vi "Principal.vi"() -> ()   [LabVIEW 2018]
uses:
  <vilib>/LabVIEW Interface for Arduino/Type Defs/Arduino Resource.ctl
  <vilib>/LabVIEW Interface for Arduino/Type Defs/Board Type.ctl
  <vilib>/LabVIEW Interface for Arduino/Type Defs/Connection Type.ctl
  <vilib>/LabVIEW Interface for Arduino/Type Defs/Pin Mode.ctl
  <vilib>/LabVIEW Interface for Arduino/LabVIEW Interface for Arduino.lvlib
panel:
  out "Mensagem":string
  in  "ATUALIZAR CAP":bool=TRUE
  in  "index":i32
  out "CAL":bool=TRUE
  out "Arduino Resource out":T3
  out "BT_Endereco":string[](array[string])
  out "BT_Nome":string[](array[string])
  in  "Frames":enum32{"Menu", "Medição", "Calibração"}(tab)
  in  "SAIR":bool
  in  "Atualizar":bool
  in  "Dispositivos Encontrados":i32(listbox)
  in  "Conectar":bool
  in  "Cap Ext.":bool
  in  "Resitor:":u32=4700 format="%.0f Ohms"
  in  "SAIR 2":bool
  in  "Capacitor:":dbl=0.8 min=0.0 max=408.8 step=0.8 format="%.2f uF"
  in  "LER CAPACITOR":bool
  out "Valor Lido:":dbl format="%.2f uF"
  in  "STOP CAL":bool
  out "Table":string[][](table)
  in  "CALIBRA敲O":bool
  out "Tempo Estimado (s)":dbl
  out "Pontos Lidos":dbl
  out "Pontos Restante":dbl
  out "Arduino Resource":T4={"VISA resource"="", "Board Type"=enum."Uno", "Connection Type"=enum."USB / Serial", "Bytes Per Packet (15)"=15}
  # "V2.1"
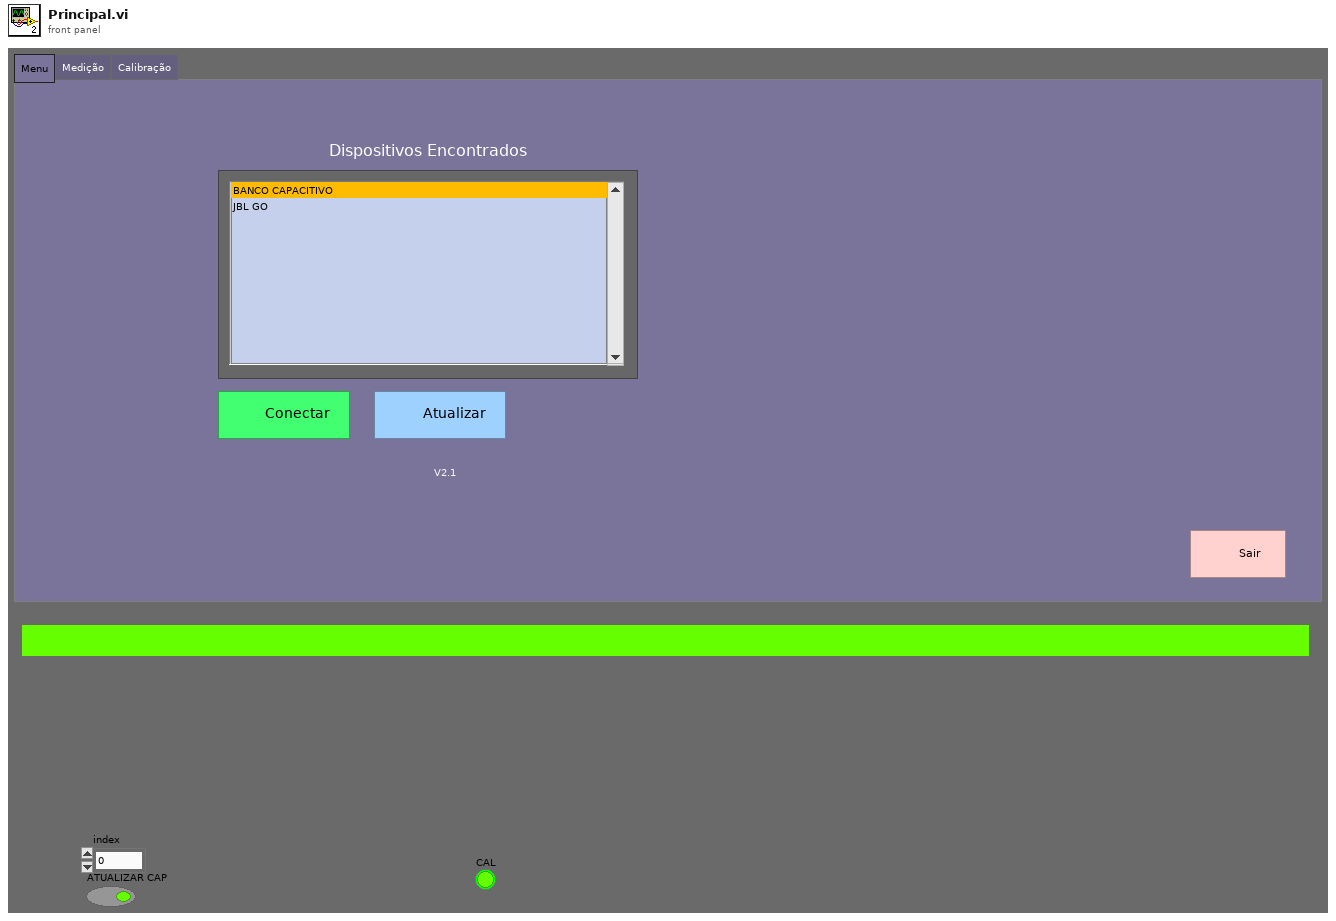
[diagram p1: front panel]
types:
  T1 = typedef "LabVIEW Interface for Arduino.lvlib/Board Type.ctl" = enum16{"Uno", "Dimuelanove w/Atmega 328", "Mega 2560"}
  T2 = typedef "LabVIEW Interface for Arduino.lvlib/Connection Type.ctl" = enum8{"USB / Serial", "XBEE", "BlueSmirf (Bluetooth)"}
  T3 = cluster{"connection ID in":refnum<k31>, "Board Type (Uno)":T1, "Connection Type (USB/Serial)":T2, "Bytes Per Packet (15)":u32}
  T4 = typedef "LabVIEW Interface for Arduino.lvlib/Arduino Resource.ctl" = cluster{"VISA resource":refnum<visa-resource-name>, "Board Type":T1, "Connection Type":enum8{"USB / Serial"}, "Bytes Per Packet (15)":u8}
  T5 = typedef "LabVIEW Interface for Arduino.lvlib/Pin Mode.ctl" = enum8{"Input", "Output"}
  T6 = cluster{"Address":string, "Device Name":string}[]
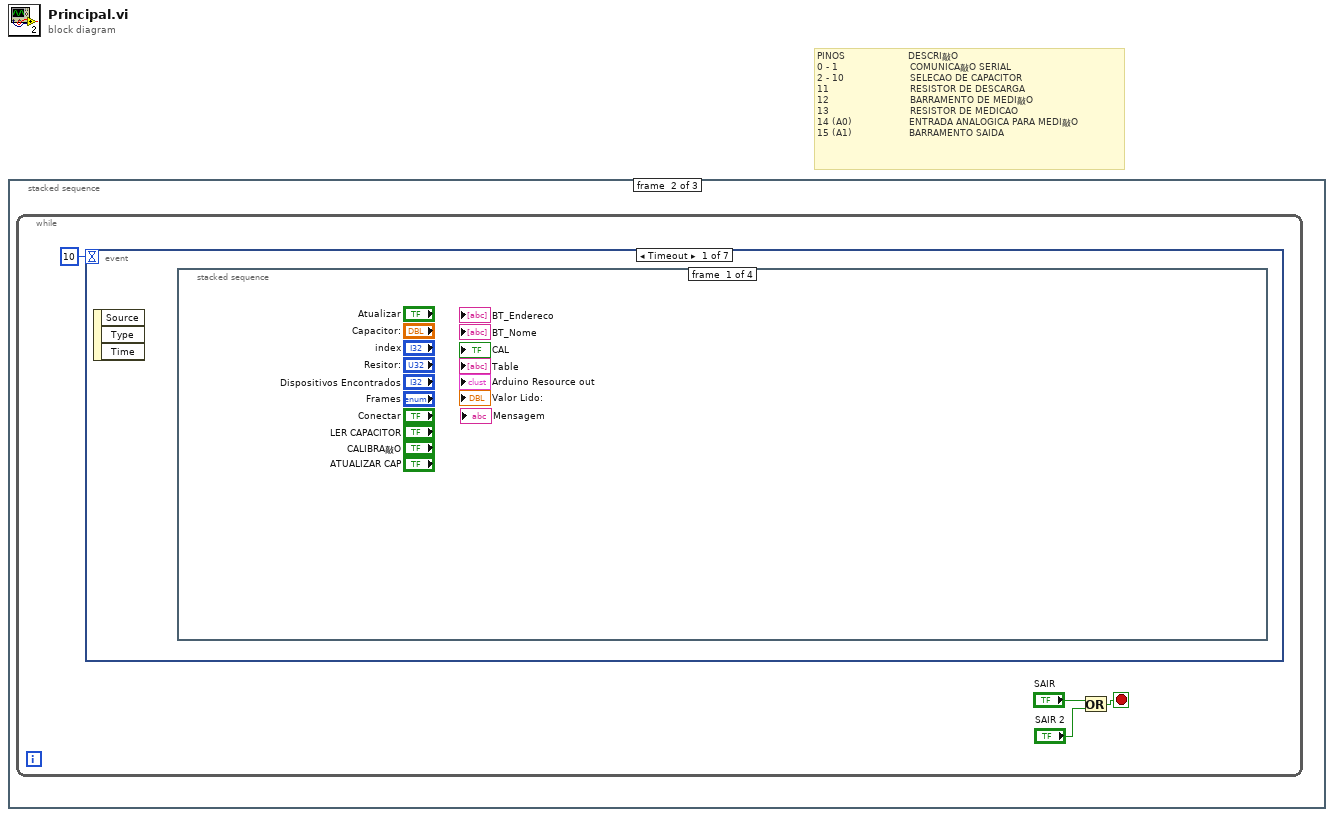
[diagram p0: block diagram]
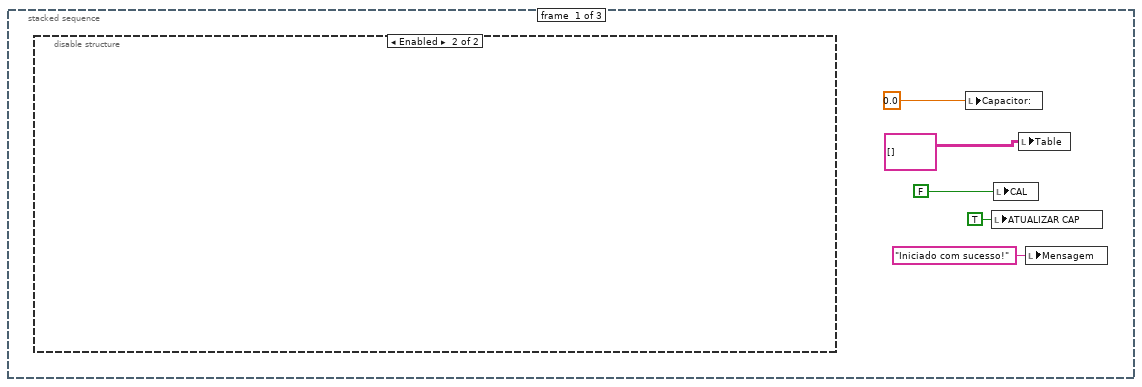
[diagram p2: hidden frame]
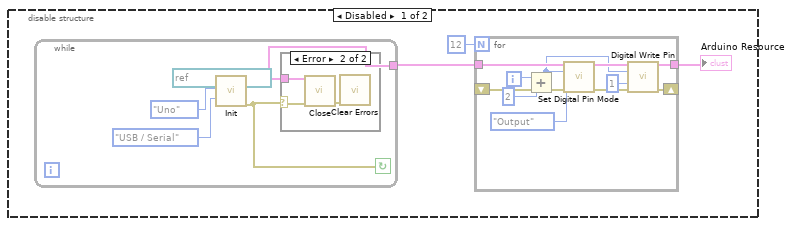
[diagram p3: hidden frame]
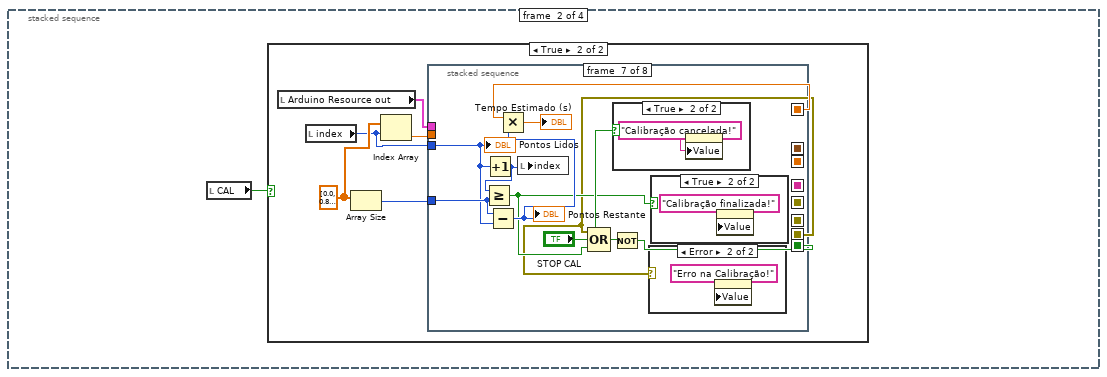
[diagram p5: hidden frame]
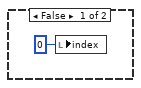
[diagram p6: hidden frame]
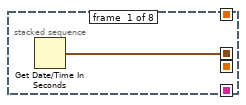
[diagram p7: hidden frame]
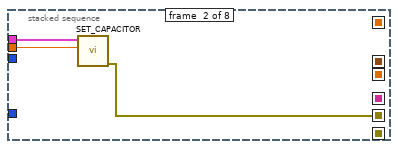
[diagram p8: hidden frame]
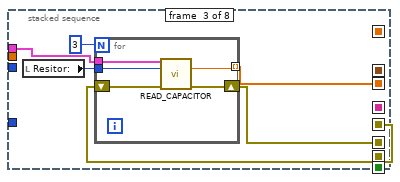
[diagram p9: hidden frame]
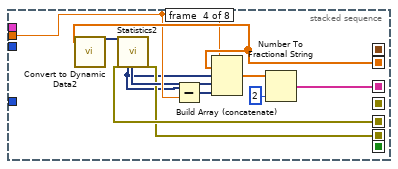
[diagram p10: hidden frame]
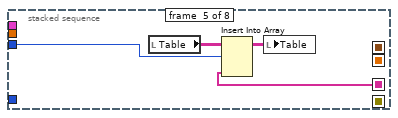
[diagram p11: hidden frame]
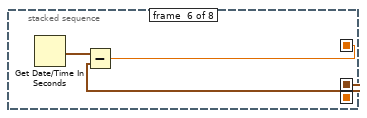
[diagram p12: hidden frame]
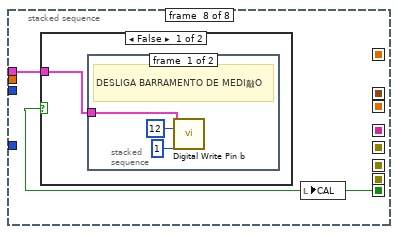
[diagram p16: hidden frame]
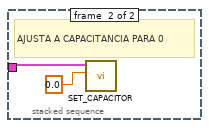
[diagram p17: hidden frame]
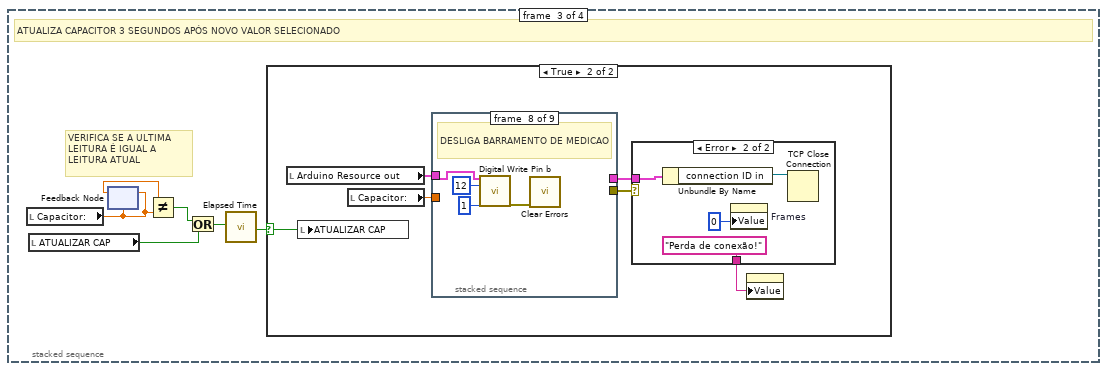
[diagram p19: hidden frame]
diagram:
  # "PINOS                     DESCRI敲O\n0 - 1                        COMUNICA敲O SERIAL\n2 - 10                      SELECAO DE CAPACITOR\n11                           RESISTOR DE DESCARGA\n12                           BARRAMENTO DE MEDI敲O\n13                           RESISTOR DE MEDICAO\n14 (A0)                   ENTRADA ANALOGICA PARA MEDI敲O\n15 (A1)                   BARRAMENTO SAIDA"
  n1 = stacked-sequence {
    frame #0 {
      n2 = disable-structure shown="Enabled" {
        frame Disabled {
          n3 = while {
            tunnel: [w21] -> w7
            stop <- w22 continue-if-true
            n4 = call <vilib>:"Init.vi"("VISA resource"=refnum<visa-resource-name> "ASRL8::INSTR", "Board Type (Uno)"=Board_Type."Uno", "Connection Type (USB/Serial)"=Connection_Type."USB / Serial") -> ("Arduino Resource"=w21:T4, "error out"=w22:errorcluster)  [unwired: 15 in]
            n5 = case shown="Error" w22 {
              selector: w22 -> [_ w26]
              tunnel: w21 -> [_ w27]
              frame No Error {
              }
              frame Error {
                n6 = call <vilib>:"Close.vi"("Arduino Resource"=w27, "error in"=w26) -> ("error out"=w25:errorcluster)  [unwired: 13 in]
                n7 = call <vilib>:"Clear Errors.vi"("error in (no error)"=w25) -> ()  [unwired: 5 in, 2 out]
              }
            }
          }
          n8 = for {
            N: 12 -> [_]
            tunnel: w7 -> [w19]
            shift-right: [w14] -> _
            shift-left: _ -> [w17]
            tunnel: [w13] -> w8
            i -> [w12]
            n9 = Add(x=w12, y=2) -> (x+y=w11:i32)
            n10 = call <vilib>:"Set Digital Pin Mode.vi"("Arduino Resource"=w19, "Digital I/O Pin"=w11, "Pin Mode (Input)"=Pin_Mode."Output", "error in"=w17) -> ("Arduino Resource"=w16:T4, "error out"=w15:errorcluster)  [unwired: 10 in]
            n11 = call <vilib>:"Digital Write Pin.vi"("Arduino Resource"=w16, "Digital I/O Pin (0)"=w11, "Value (0)"=u8 1, "error in"=w15) -> ("Arduino Resource"=w13:T4, "error out"=w14:errorcluster)  [unwired: 10 in]
          }
          "Arduino Resource" <- w8
        }
        frame Enabled {
        }
      }
      n12 = local write "Capacitor:"(0.0 ("Capacitor")) -> ()
      n13 = local write "ATUALIZAR CAP"(TRUE ("ATUALIZAR CAP")) -> ()
      n14 = local write "CAL"(FALSE ("CAL")) -> ()
      n15 = local write "Table"(string[][] [] ("Table")) -> ()
      n16 = local write "Mensagem"("Iniciado com sucesso!" ("Mensagem")) -> ()
    }
    frame #1 {
      n17 = while {
        stop <- w28 stop-if-true
        n18 = event shown="[0] Timeout" {
          selector: _ -> [_ _ _ _ _ _ _]
          dyn-events: _ -> [_ _ _ _ _ _ _]
          timeout: 10 -> [_ _ _ _ _ _ _]
          event Timeout {
            n19 = event-data() -> ()  [unwired: 1 in, 3 out]
            n20 = stacked-sequence {
              frame #0 {
              }
              frame #1 {
                n21 = local read "CAL"() -> (w32:bool)
                n22 = case shown="True" w32 {
                  frame False {
                    n23 = local write "index"(0 ("index")) -> ()
                  }
                  frame True {
                    w37 = dbl[] [0.0, 0.8, 1.6, 2.4000000000000004, 3.2, 4.0, 4.8, 5.6, 6.3999999999999995, 7.199999999999999, 7.999999999999999, 8.799999999999999, 9.6, 10.4, 11.200000000000001, 12.000000000000002, 12.800000000000002, 13.600000000000003, 14.400000000000004, 15.200000000000005, 16.000000000000004, 16.800000000000004, 17.600000000000005, 18.400000000000006, 19.200000000000006, 20.000000000000007, 20.800000000000008, 21.60000000000001, 22.40000000000001, 23.20000000000001, 24.00000000000001, 24.80000000000001, 25.600000000000012, 26.400000000000013, 27.200000000000014, 28.000000000000014, 28.800000000000015, 29.600000000000016, 30.400000000000016, 31.200000000000017, 32.000000000000014, 32.80000000000001, 33.60000000000001, 34.400000000000006, 35.2, 36.0, 36.8, 37.599999999999994, 38.39999999999999, 39.19999999999999, 39.999999999999986, 40.79999999999998, 41.59999999999998, 42.39999999999998, 43.199999999999974, 43.99999999999997, 44.79999999999997, 45.599999999999966, 46.39999999999996, 47.19999999999996, 47.99999999999996, 48.799999999999955, 49.59999999999995, 50.39999999999995, 51.199999999999946, 51.99999999999994, 52.79999999999994, 53.59999999999994, 54.399999999999935, 55.19999999999993, 55.99999999999993, 56.799999999999926, 57.59999999999992, 58.39999999999992, 59.19999999999992, 59.999999999999915, 60.79999999999991, 61.59999999999991, 62.399999999999906, 63.1999999999999, 63.9999999999999, 64.7999999999999, 65.5999999999999, 66.39999999999989, 67.19999999999989, 67.99999999999989, 68.79999999999988, 69.59999999999988, 70.39999999999988, 71.19999999999987, 71.99999999999987, 72.79999999999987, 73.59999999999987, 74.39999999999986, 75.19999999999986, 75.99999999999986, 76.79999999999986, 77.59999999999985, 78.39999999999985, 79.19999999999985, 79.99999999999984, 80.79999999999984, 81.59999999999984, 82.39999999999984, 83.19999999999983, 83.99999999999983, 84.79999999999983, 85.59999999999982, 86.39999999999982, 87.19999999999982, 87.99999999999982, 88.79999999999981, 89.59999999999981, 90.3999999999998, 91.1999999999998, 91.9999999999998, 92.7999999999998, 93.5999999999998, 94.39999999999979, 95.19999999999979, 95.99999999999979, 96.79999999999978, 97.59999999999978, 98.39999999999978, 99.19999999999978, 99.99999999999977, 100.79999999999977, 101.59999999999977, 102.39999999999976, 103.19999999999976, 103.99999999999976, 104.79999999999976, 105.59999999999975, 106.39999999999975, 107.19999999999975, 107.99999999999974, 108.79999999999974, 109.59999999999974, 110.39999999999974, 111.19999999999973, 111.99999999999973, 112.79999999999973, 113.59999999999972, 114.39999999999972, 115.19999999999972, 115.99999999999972, 116.79999999999971, 117.59999999999971, 118.39999999999971, 119.1999999999997, 119.9999999999997, 120.7999999999997, 121.5999999999997, 122.3999999999997, 123.19999999999969, 123.99999999999969, 124.79999999999968, 125.59999999999968, 126.39999999999968, 127.19999999999968, 127.99999999999967, 128.79999999999967, 129.59999999999968, 130.3999999999997, 131.1999999999997, 131.99999999999972, 132.79999999999973, 133.59999999999974, 134.39999999999975, 135.19999999999976, 135.99999999999977, 136.79999999999978, 137.5999999999998, 138.3999999999998, 139.19999999999982, 139.99999999999983, 140.79999999999984, 141.59999999999985, 142.39999999999986, 143.19999999999987, 143.9999999999999, 144.7999999999999, 145.5999999999999, 146.39999999999992, 147.19999999999993, 147.99999999999994, 148.79999999999995, 149.59999999999997, 150.39999999999998, 151.2, 152.0, 152.8, 153.60000000000002, 154.40000000000003, 155.20000000000005, 156.00000000000006, 156.80000000000007, 157.60000000000008, 158.4000000000001, 159.2000000000001, 160.0000000000001, 160.80000000000013, 161.60000000000014, 162.40000000000015, 163.20000000000016, 164.00000000000017, 164.80000000000018, 165.6000000000002, 166.4000000000002, 167.20000000000022, 168.00000000000023, 168.80000000000024, 169.60000000000025, 170.40000000000026, 171.20000000000027, 172.00000000000028, 172.8000000000003, 173.6000000000003, 174.40000000000032, 175.20000000000033, 176.00000000000034, 176.80000000000035, 177.60000000000036, 178.40000000000038, 179.2000000000004, 180.0000000000004, 180.8000000000004, 181.60000000000042, 182.40000000000043, 183.20000000000044, 184.00000000000045, 184.80000000000047, 185.60000000000048, 186.4000000000005, 187.2000000000005, 188.0000000000005, 188.80000000000052, 189.60000000000053, 190.40000000000055, 191.20000000000056, 192.00000000000057, 192.80000000000058, 193.6000000000006, 194.4000000000006, 195.2000000000006, 196.00000000000063, 196.80000000000064, 197.60000000000065, 198.40000000000066, 199.20000000000067, 200.00000000000068, 200.8000000000007, 201.6000000000007, 202.40000000000072, 203.20000000000073, 204.00000000000074, 204.80000000000075, 205.60000000000076, 206.40000000000077, 207.20000000000078, 208.0000000000008, 208.8000000000008, 209.60000000000082, 210.40000000000083, 211.20000000000084, 212.00000000000085, 212.80000000000086, 213.60000000000088, 214.4000000000009, 215.2000000000009, 216.0000000000009, 216.80000000000092, 217.60000000000093, 218.40000000000094, 219.20000000000095, 220.00000000000097, 220.80000000000098, 221.600000000001, 222.400000000001, 223.200000000001, 224.00000000000102, 224.80000000000103, 225.60000000000105, 226.40000000000106, 227.20000000000107, 228.00000000000108, 228.8000000000011, 229.6000000000011, 230.4000000000011, 231.20000000000113, 232.00000000000114, 232.80000000000115, 233.60000000000116, 234.40000000000117, 235.20000000000118, 236.0000000000012, 236.8000000000012, 237.60000000000122, 238.40000000000123, 239.20000000000124, 240.00000000000125, 240.80000000000126, 241.60000000000127, 242.40000000000128, 243.2000000000013, 244.0000000000013, 244.80000000000132, 245.60000000000133, 246.40000000000134, 247.20000000000135, 248.00000000000136, 248.80000000000138, 249.6000000000014, 250.4000000000014, 251.2000000000014, 252.00000000000142, 252.80000000000143, 253.60000000000144, 254.40000000000146, 255.20000000000147, 256.0000000000015, 256.8000000000015, 257.6000000000015, 258.4000000000015, 259.2000000000015, 260.00000000000153, 260.80000000000155, 261.60000000000156, 262.40000000000157, 263.2000000000016, 264.0000000000016, 264.8000000000016, 265.6000000000016, 266.4000000000016, 267.20000000000164, 268.00000000000165, 268.80000000000166, 269.60000000000167, 270.4000000000017, 271.2000000000017, 272.0000000000017, 272.8000000000017, 273.6000000000017, 274.40000000000174, 275.20000000000175, 276.00000000000176, 276.8000000000018, 277.6000000000018, 278.4000000000018, 279.2000000000018, 280.0000000000018, 280.80000000000183, 281.60000000000184, 282.40000000000185, 283.20000000000186, 284.0000000000019, 284.8000000000019, 285.6000000000019, 286.4000000000019, 287.2000000000019, 288.00000000000193, 288.80000000000194, 289.60000000000196, 290.40000000000197, 291.200000000002, 292.000000000002, 292.800000000002, 293.600000000002, 294.400000000002, 295.20000000000203, 296.00000000000205, 296.80000000000206, 297.60000000000207, 298.4000000000021, 299.2000000000021, 300.0000000000021, 300.8000000000021, 301.6000000000021, 302.40000000000214, 303.20000000000215, 304.00000000000216, 304.80000000000217, 305.6000000000022, 306.4000000000022, 307.2000000000022, 308.0000000000022, 308.8000000000022, 309.60000000000224, 310.40000000000225, 311.20000000000226, 312.0000000000023, 312.8000000000023, 313.6000000000023, 314.4000000000023, 315.2000000000023, 316.00000000000233, 316.80000000000234, 317.60000000000235, 318.40000000000236, 319.2000000000024, 320.0000000000024, 320.8000000000024, 321.6000000000024, 322.4000000000024, 323.20000000000243, 324.00000000000244, 324.80000000000246, 325.60000000000247, 326.4000000000025, 327.2000000000025, 328.0000000000025, 328.8000000000025, 329.6000000000025, 330.40000000000254, 331.20000000000255, 332.00000000000256, 332.80000000000257, 333.6000000000026, 334.4000000000026, 335.2000000000026, 336.0000000000026, 336.8000000000026, 337.60000000000264, 338.40000000000265, 339.20000000000266, 340.0000000000027, 340.8000000000027, 341.6000000000027, 342.4000000000027, 343.2000000000027, 344.00000000000273, 344.80000000000274, 345.60000000000275, 346.40000000000276, 347.2000000000028, 348.0000000000028, 348.8000000000028, 349.6000000000028, 350.4000000000028, 351.20000000000283, 352.00000000000284, 352.80000000000285, 353.60000000000286, 354.4000000000029, 355.2000000000029, 356.0000000000029, 356.8000000000029, 357.6000000000029, 358.40000000000293, 359.20000000000294, 360.00000000000296, 360.80000000000297, 361.600000000003, 362.400000000003, 363.200000000003, 364.000000000003, 364.800000000003, 365.60000000000304, 366.40000000000305, 367.20000000000306, 368.00000000000307, 368.8000000000031, 369.6000000000031, 370.4000000000031, 371.2000000000031, 372.0000000000031, 372.80000000000314, 373.60000000000315, 374.40000000000316, 375.2000000000032, 376.0000000000032, 376.8000000000032, 377.6000000000032, 378.4000000000032, 379.20000000000323, 380.00000000000324, 380.80000000000325, 381.60000000000326, 382.4000000000033, 383.2000000000033, 384.0000000000033, 384.8000000000033, 385.6000000000033, 386.40000000000333, 387.20000000000334, 388.00000000000335, 388.80000000000337, 389.6000000000034, 390.4000000000034, 391.2000000000034, 392.0000000000034, 392.8000000000034, 393.60000000000343, 394.40000000000344, 395.20000000000346, 396.00000000000347, 396.8000000000035, 397.6000000000035, 398.4000000000035, 399.2000000000035, 400.0000000000035, 400.80000000000354, 401.60000000000355, 402.40000000000356, 403.20000000000357, 404.0000000000036, 404.8000000000036, 405.6000000000036, 406.4000000000036, 407.2000000000036, 408.00000000000364, 408.80000000000365] ("Array")
                    n24 = local read "Arduino Resource out"() -> (w38:T3)
                    n25 = local read "index"() -> (w35:i32)
                    n26 = Array Size(array=w37) -> (size(s)=w34:i32)
                    n27 = Index Array(array=w37, index=w35) -> (element=w36:dbl)
                    n28 = stacked-sequence {
                      seq-local: [w39 _ _ _ _ _ _ _] -> [_ _ _ _ _ w70 _ _]
                      seq-local: [_ _ w45 _ _ _ _ _] -> [_ _ _ w63 _ _ _ _]
                      seq-local: [_ _ _ w60 _ _ _ _] -> [_ _ _ _ w66 _ _ _]
                      seq-local: [_ w40 _ _ _ _ _ _] -> [_ _ w44 _ _ _ _ _]
                      seq-local: [_ _ w43 _ _ _ _ _] -> [_ _ _ w59 _ _ _ _]
                      seq-local: [_ _ _ _ _ w69 _ _] -> [_ _ _ _ _ _ w78 _]
                      seq-local: [_ _ _ w55 _ _ _ _] -> [_ _ _ _ _ _ w73 _]
                      seq-local: [_ _ _ _ _ _ w76 _] -> [_ _ _ _ _ _ _ w87]
                      tunnel: w35 -> [_ _ _ _ w65 _ w80 _]
                      tunnel: w36 -> [_ w41 _ w58 _ _ _ _]
                      tunnel: w38 -> [_ w42 w46 _ _ _ _ w86]
                      tunnel: w34 -> [_ _ _ _ _ _ w81 _]
                      frame #0 {
                        n29 = Get Date/Time In Seconds() -> (seconds since 1Jan1904=w39:timestamp)
                      }
                      frame #1 {
                        n30 = call "SET_CAPACITOR.vi"("Arduino Resource in"=w42, "Capacitor"=w41) -> ("error out"=w40:errorcluster)  [unwired: 7 in, 1 out]
                      }
                      frame #2 {
                        n31 = local read "Resitor:"() -> (w48:u32)
                        n32 = for {
                          N: 3 -> [_]
                          tunnel: w46 -> [w52]
                          tunnel: w48 -> [w51]
                          tunnel: [w50] -> w45 mode=indexing
                          shift-right: [w49] -> w43
                          shift-left: w44 -> [w53]
                          n33 = call "READ_CAPACITOR.vi"("Arduino Resource in"=w52, "Resitor"=w51, "error in"=w53) -> ("Capacitor"=w50:dbl, "error out"=w49:errorcluster)  [unwired: 10 in, 1 out]
                        }
                      }
                      frame #3 {
                        n34 = call "Convert to Dynamic Data2"("Array"=w63) -> ("Dynamic Data Type"=w64:dynamicdata)  [unwired: 3 in]
                        n35 = call "Statistics2"("Signals"=w64, "error in (no error)"=w59) -> ("Median"=w54:dynamicdata, "Standard Dev"=w56:dynamicdata, "error out"=w55:errorcluster)  [unwired: 23 in]
                        n36 = Subtract(x=w54, y=w58) -> (x-y=w57:dynamicdata)
                        n37 = Build Array (concatenate)(w58, w63, w54, w56, w57) -> (w62:dbl[])
                        n38 = Number To Fractional String(number=w62, precision (6)=i16 2) -> (F-format string=w60:string[])  [unwired: 2 in]
                      }
                      frame #4 {
                        n39 = local read "Table"() -> (w68:string[][])
                        n40 = Insert Into Array(array=w68, index (row)=w65, new element=w66) -> (w67:string[][])  [unwired: 1 in]
                        n41 = local write "Table"(w67) -> ()
                      }
                      frame #5 {
                        n42 = Get Date/Time In Seconds() -> (seconds since 1Jan1904=w71:timestamp)
                        n43 = Subtract(x=w71, y=w70) -> (x-y=w69:dbl)
                      }
                      frame #6 {
                        n44 = Increment(x=w80) -> (x+1=w82:i32)
                        n45 = Greater Or Equal?(x=w82, y=w81) -> (x >= y?=w74:bool)
                        n46 = Subtract(x=w81, y=w80) -> (x-y=w79:i32)
                        "Pontos Restante" <- w79
                        n47 = Multiply(x=w78, y=w79) -> (x*y=→"Tempo Estimado (s)":dbl)
                        n48 = local write "index"(w82) -> ()
                        n49 = Compound Arithmetic op=OR(w73, "STOP CAL", w74) -> (w77:bool)
                        n50 = Not(x=w77) -> (.not. x?=w76:bool)
                        n51 = case shown="True" "STOP CAL" {
                          frame False {
                          }
                          frame True {
                            n52 = property on="Mensagem" class="Str"("Value"="Calibração cancelada!" ("Mensagem")) -> ()  [unwired: 2 in, 2 out]
                          }
                        }
                        n53 = case shown="Error" w73 {
                          frame No Error {
                          }
                          frame Error {
                            n54 = property on="Mensagem" class="Str"("Value"="Erro na Calibração!" ("Mensagem")) -> ()  [unwired: 2 in, 2 out]
                          }
                        }
                        n55 = case shown="True" w74 {
                          frame False {
                          }
                          frame True {
                            n56 = property on="Mensagem" class="Str"("Value"="Calibração finalizada!" ("Mensagem")) -> ()  [unwired: 2 in, 2 out]
                          }
                        }
                        "Pontos Lidos" <- w80
                      }
                      frame #7 {
                        n57 = case shown="False" w87 {
                          tunnel: w86 -> [w88 _]
                          frame False {
                            n58 = stacked-sequence {
                              tunnel: w88 -> [w89 w93]
                              frame #0 {
                                # "DESLIGA BARRAMENTO DE MEDI敲O"
                                n59 = call "Digital Write Pin b.vi"("Arduino Resource in"=w89, "Digital I/O Pin (0)"=u8 12, "Value (0)"=u8 1) -> ()  [unwired: 11 in, 2 out]
                              }
                              frame #1 {
                                # "AJUSTA A CAPACITANCIA PARA 0"
                                n60 = call "SET_CAPACITOR.vi"("Arduino Resource in"=w93, "Capacitor"=0.0) -> ()  [unwired: 7 in, 2 out]
                              }
                            }
                          }
                          frame True {
                          }
                        }
                        n61 = local write "CAL"(w87) -> ()
                      }
                    }
                  }
                }
              }
              frame #2 {
                # "VERIFICA SE A ULTIMA \nLEITURA É IGUAL A \nLEITURA ATUAL"
                # "ATUALIZA CAPACITOR 3 SEGUNDOS APÓS NOVO VALOR SELECIONADO"
                n62 = local read "Capacitor:"() -> (w95:dbl)
                n63 = local read "ATUALIZAR CAP"() -> (w98:bool)
                n64 = feedback-in #1(w95) -> ()
                n65 = feedback #1(w95) -> (w96:dbl)
                n66 = Not Equal?(x=w96, y=w95) -> (x != y?=w94:bool)
                n67 = Or(x=w94, y=w98) -> (x .or. y?=w97:bool)
                n68 = call "Elapsed Time"("Reset"=w97) -> ("Time has Elapsed"=w99:bool)  [unwired: 11 in, 7 out]
                n69 = case shown="True" w99 {
                  selector: w99 -> [_ w101]
                  frame False {
                  }
                  frame True {
                    n70 = local read "Arduino Resource out"() -> (w103:T3)
                    n71 = local write "ATUALIZAR CAP"(w101) -> ()
                    n72 = local read "Capacitor:"() -> (w105:dbl)
                    n73 = stacked-sequence {
                      tunnel: w103 -> [w109 w114 _ w118 w120 w125 w130 w132 w137]
                      tunnel: w105 -> [_ _ _ w117 _ _ _ _ _]
                      tunnel: [_ _ _ _ _ _ _ _ w136] -> w104
                      tunnel: [_ _ _ _ _ _ _ _ w135] -> w102
                      frame #0 {
                        # "DESLIGA BARRAMENTO"
                        n74 = call "Digital Write Pin b.vi"("Arduino Resource in"=w109, "Digital I/O Pin (0)"=u8 15, "Value (0)"=u8 1) -> ("error out"=w106:errorcluster)  [unwired: 11 in, 1 out]
                        n75 = call <vilib>:"Clear Errors.vi"("error in (no error)"=w106) -> ()  [unwired: 5 in, 2 out]
                      }
                      frame #1 {
                        # "LIGA RESITOR DE DESCARGA"
                        n76 = call "Digital Write Pin b.vi"("Arduino Resource in"=w114, "Digital I/O Pin (0)"=u8 11, "Value (0)"=u8 0) -> ("error out"=w111:errorcluster)  [unwired: 11 in, 1 out]
                        n77 = call <vilib>:"Clear Errors.vi"("error in (no error)"=w111) -> ()  [unwired: 5 in, 2 out]
                        n78 = property on="Mensagem" class="Str"("Value"="Descarregando Capacitores!" ("Mensagem")) -> ()  [unwired: 2 in, 2 out]
                      }
                      frame #2 {
                        # "AGUARDA DESCARGA"
                        n79 = Wait (ms)(milliseconds to wait=u32 3000) -> ()  [unwired: 1 out]
                      }
                      frame #3 {
                        # "AJUSTA VALOR DO CAPACITOR"
                        n80 = call "SET_CAPACITOR.vi"("Arduino Resource in"=w118, "Capacitor"=w117) -> ("error out"=w116:errorcluster)  [unwired: 7 in, 1 out]
                        n81 = call <vilib>:"Clear Errors.vi"("error in (no error)"=w116) -> ()  [unwired: 5 in, 2 out]
                      }
                      frame #4 {
                        # "DESLIGA RESISTOR DE DESCARGA"
                        n82 = call "Digital Write Pin b.vi"("Arduino Resource in"=w120, "Digital I/O Pin (0)"=u8 11, "Value (0)"=u8 1) -> ("error out"=w119:errorcluster)  [unwired: 11 in, 1 out]
                        n83 = call <vilib>:"Clear Errors.vi"("error in (no error)"=w119) -> ()  [unwired: 5 in, 2 out]
                      }
                      frame #5 {
                        # "LIGA BARRAMENTO DE MEDI敲O"
                        n84 = call "Digital Write Pin b.vi"("Arduino Resource in"=w125, "Digital I/O Pin (0)"=u8 12, "Value (0)"=u8 0) -> ("error out"=w124:errorcluster)  [unwired: 11 in, 1 out]
                        n85 = property on="Mensagem" class="Str"("Value"="Medindo capacitor!" ("Mensagem")) -> ()  [unwired: 2 in, 2 out]
                        n86 = call <vilib>:"Clear Errors.vi"("error in (no error)"=w124) -> ()  [unwired: 5 in, 2 out]
                      }
                      frame #6 {
                        # "EXECUTA MEDI敲O"
                        n87 = call "READ_CAPACITOR.vi"("Arduino Resource in"=w130) -> ("Capacitor"=w129:dbl, "error out"=w128:errorcluster)  [unwired: 12 in, 1 out]
                        n88 = local write "Valor Lido:"(w129) -> ()
                        n89 = call <vilib>:"Clear Errors.vi"("error in (no error)"=w128) -> ()  [unwired: 5 in, 2 out]
                      }
                      frame #7 {
                        # "DESLIGA BARRAMENTO DE MEDICAO"
                        n90 = call "Digital Write Pin b.vi"("Arduino Resource in"=w132, "Digital I/O Pin (0)"=u8 12, "Value (0)"=u8 1) -> ("error out"=w131:errorcluster)  [unwired: 11 in, 1 out]
                        n91 = call <vilib>:"Clear Errors.vi"("error in (no error)"=w131) -> ()  [unwired: 5 in, 2 out]
                      }
                      frame #8 {
                        # "LIGA BARRAMENTO SAIDA"
                        n92 = call "Digital Write Pin b.vi"("Arduino Resource in"=w137, "Digital I/O Pin (0)"=u8 15, "Value (0)"=u8 0) -> ("Arduino Resource out"=w135:T3, "error out"=w136:errorcluster)  [unwired: 11 in]
                      }
                    }
                    n93 = case shown="Error" w104 {
                      tunnel: w102 -> [_ w145]
                      tunnel: ["Capacitor atualizado!" ("Mensagem") "Perda de conexão!" ("Mensagem")] -> w100
                      frame No Error {
                        n94 = property on="Frames" class="TabCtl (strict)"("Value"=u8 1 ("Value (0)")) -> ()  [unwired: 2 in, 2 out]
                      }
                      frame Error {
                        n95 = Unbundle By Name(w145) -> ("connection ID in"=w144:refnum<k31>)
                        n96 = property on="Frames" class="TabCtl (strict)"("Value"=u8 0 ("Value (0)")) -> ()  [unwired: 2 in, 2 out]
                        n97 = TCP Close Connection(connection ID=w144) -> ()  [unwired: 2 in, 2 out]
                      }
                    }
                    n98 = property on="Mensagem" class="Str"("Value"=w100) -> ()  [unwired: 2 in, 2 out]
                  }
                }
              }
              frame #3 {
                # "LE CAPACITOR EXTERNO"
                n99 = case shown="True" "Cap Ext." {
                  frame False {
                  }
                  frame True {
                    n100 = local read "Arduino Resource out"() -> (w150:T3)
                    n101 = stacked-sequence {
                      tunnel: w150 -> [w155 w160 _ w164 w166 w171 w176 w178 w183 w186]
                      tunnel: 0.0 ("Capacitor:") -> [_ _ _ w163 _ _ _ _ _ _]
                      tunnel: [_ _ _ _ _ _ _ _ w182 _] -> w151
                      tunnel: [_ _ _ _ _ _ _ _ w181 _] -> w149
                      frame #0 {
                        # "DESLIGA BARRAMENTO"
                        n102 = call "Digital Write Pin b.vi"("Arduino Resource in"=w155, "Digital I/O Pin (0)"=u8 15, "Value (0)"=u8 1) -> ("error out"=w152:errorcluster)  [unwired: 11 in, 1 out]
                        n103 = call <vilib>:"Clear Errors.vi"("error in (no error)"=w152) -> ()  [unwired: 5 in, 2 out]
                      }
                      frame #1 {
                        # "LIGA RESITOR DE DESCARGA"
                        n104 = call "Digital Write Pin b.vi"("Arduino Resource in"=w160, "Digital I/O Pin (0)"=u8 11, "Value (0)"=u8 0) -> ("error out"=w157:errorcluster)  [unwired: 11 in, 1 out]
                        n105 = call <vilib>:"Clear Errors.vi"("error in (no error)"=w157) -> ()  [unwired: 5 in, 2 out]
                        n106 = property on="Mensagem" class="Str"("Value"="Descarregando Capacitores!" ("Mensagem")) -> ()  [unwired: 2 in, 2 out]
                      }
                      frame #2 {
                        # "AGUARDA DESCARGA"
                        n107 = Wait (ms)(milliseconds to wait=u32 3000) -> ()  [unwired: 1 out]
                      }
                      frame #3 {
                        # "AJUSTA VALOR DO CAPACITOR"
                        n108 = call "SET_CAPACITOR.vi"("Arduino Resource in"=w164, "Capacitor"=w163) -> ("error out"=w162:errorcluster)  [unwired: 7 in, 1 out]
                        n109 = call <vilib>:"Clear Errors.vi"("error in (no error)"=w162) -> ()  [unwired: 5 in, 2 out]
                      }
                      frame #4 {
                        # "DESLIGA RESISTOR DE DESCARGA"
                        n110 = call "Digital Write Pin b.vi"("Arduino Resource in"=w166, "Digital I/O Pin (0)"=u8 11, "Value (0)"=u8 1) -> ("error out"=w165:errorcluster)  [unwired: 11 in, 1 out]
                        n111 = call <vilib>:"Clear Errors.vi"("error in (no error)"=w165) -> ()  [unwired: 5 in, 2 out]
                      }
                      frame #5 {
                        # "LIGA BARRAMENTO DE MEDI敲O"
                        n112 = call "Digital Write Pin b.vi"("Arduino Resource in"=w171, "Digital I/O Pin (0)"=u8 12, "Value (0)"=u8 0) -> ("error out"=w170:errorcluster)  [unwired: 11 in, 1 out]
                        n113 = property on="Mensagem" class="Str"("Value"="Medindo capacitor externo!" ("Mensagem")) -> ()  [unwired: 2 in, 2 out]
                        n114 = call <vilib>:"Clear Errors.vi"("error in (no error)"=w170) -> ()  [unwired: 5 in, 2 out]
                      }
                      frame #6 {
                        # "EXECUTA MEDI敲O"
                        n115 = call "READ_CAPACITOR.vi"("Arduino Resource in"=w176) -> ("Capacitor"=w175:dbl, "error out"=w174:errorcluster)  [unwired: 12 in, 1 out]
                        n116 = local write "Valor Lido:"(w175) -> ()
                        n117 = call <vilib>:"Clear Errors.vi"("error in (no error)"=w174) -> ()  [unwired: 5 in, 2 out]
                      }
                      frame #7 {
                        # "DESLIGA BARRAMENTO DE MEDICAO"
                        n118 = call "Digital Write Pin b.vi"("Arduino Resource in"=w178, "Digital I/O Pin (0)"=u8 12, "Value (0)"=u8 1) -> ("error out"=w177:errorcluster)  [unwired: 11 in, 1 out]
                        n119 = call <vilib>:"Clear Errors.vi"("error in (no error)"=w177) -> ()  [unwired: 5 in, 2 out]
                      }
                      frame #8 {
                        # "LIGA BARRAMENTO SAIDA"
                        n120 = call "Digital Write Pin b.vi"("Arduino Resource in"=w183, "Digital I/O Pin (0)"=u8 15, "Value (0)"=u8 0) -> ("Arduino Resource out"=w181:T3, "error out"=w182:errorcluster)  [unwired: 11 in]
                      }
                      frame #9 {
                        # "Volta o valor dos capacitores"
                        n121 = local read "Capacitor:"() -> (w187:dbl)
                        n122 = call "SET_CAPACITOR.vi"("Arduino Resource in"=w186, "Capacitor"=w187) -> ("error out"=w188:errorcluster)  [unwired: 7 in, 1 out]
                        n123 = call <vilib>:"Clear Errors.vi"("error in (no error)"=w188) -> ()  [unwired: 5 in, 2 out]
                      }
                    }
                    n124 = case shown="No Error" w151 {
                      tunnel: w149 -> [_ w194]
                      tunnel: ["Capacitor externo medido!" ("Mensagem") "Perda de conexão!" ("Mensagem")] -> w148
                      frame No Error {
                        n125 = property on="Frames" class="TabCtl (strict)"("Value"=u8 1 ("Value (0)")) -> ()  [unwired: 2 in, 2 out]
                      }
                      frame Error {
                        n126 = Unbundle By Name(w194) -> ("connection ID in"=w193:refnum<k31>)
                        n127 = property on="Frames" class="TabCtl (strict)"("Value"=u8 0 ("Value (0)")) -> ()  [unwired: 2 in, 2 out]
                        n128 = TCP Close Connection(connection ID=w193) -> ()  [unwired: 2 in, 2 out]
                      }
                    }
                    n129 = property on="Mensagem" class="Str"("Value"=w148) -> ()  [unwired: 2 in, 2 out]
                  }
                }
              }
            }
          }
          event "Cap Ext.": Value Change {
            n130 = event-data() -> ()  [unwired: 1 in, 6 out]
          }
          event "LER CAPACITOR": Value Change {
            n131 = event-data() -> ()  [unwired: 1 in, 6 out]
            n132 = local read "Arduino Resource out"() -> (w196:T3)
            n133 = call "READ_CAPACITOR.vi"("Arduino Resource in"=w196) -> ("Capacitor"=w195:dbl)  [unwired: 12 in, 2 out]
            n134 = local write "Valor Lido:"(w195) -> ()
          }
          event "Atualizar": Value Change {
            n135 = event-data() -> ()  [unwired: 1 in, 6 out]
            n136 = Bluetooth Discover() -> (2:w204:T6)  [unwired: 2 in, 2 out]
            n137 = local write "Mensagem"("Procurando..." ("Mensagem")) -> ()
            n138 = for {
              tunnel: w204 -> [w207] mode=indexing
              tunnel: [w206] -> w203 mode=indexing
              tunnel: [w205] -> w201 mode=indexing
              n139 = Unbundle By Name(w207) -> ("Address"=w206:string, "Device Name"=w205:string)
            }
            n140 = local write "BT_Endereco"(w203) -> ()
            n141 = local write "BT_Nome"(w201) -> ()
            n142 = Array Size(array=w201) -> (size(s)=w200:i32)
            n143 = property on="Dispositivos Encontrados" class="LstBox (strict)"("Item Names"=w201) -> ()  [unwired: 2 in, 2 out]
            n144 = Number To Decimal String(number=w200) -> (decimal integer string=w199:string)  [unwired: 1 in]
            n145 = Concatenate Strings(w199, " dispositivo(s) encontrado(s)!" ("string")) -> (w197:string)
            n146 = property on="Mensagem" class="Str"("Value"=w197) -> ()  [unwired: 2 in, 2 out]
          }
          event "Conectar": Value Change {
            n147 = event-data() -> ()  [unwired: 1 in, 6 out]
            n148 = stacked-sequence {
              seq-local: [_ _ w210 _] -> [_ _ _ w257]
              frame #0 {
                n149 = Wait (ms)(milliseconds to wait=u32 100) -> ()  [unwired: 1 out]
              }
              frame #1 {
                n150 = property on="Mensagem" class="Str"("Value"="Conectando..." ("Mensagem")) -> ()  [unwired: 2 in, 2 out]
              }
              frame #2 {
                n151 = local read "BT_Endereco"() -> (w216:string[])
                n152 = property on="Dispositivos Encontrados" class="LstBox (strict)"() -> ("Value"=w215:i32)  [unwired: 2 in, 2 out]
                n153 = call "CONEXAO_BT.vi"("index"=w215, "Endereço_Lista"=w216) -> ("error out"=w213:errorcluster, "connection ID"=w214:refnum<k31>)  [unwired: 8 in]
                n154 = call "Init b.vi"("connection ID in"=w214, "Bytes Per Packet (15)"=u32 5, "error in"=w213) -> ("Arduino Resource out"=w220:T3, "error out"=w219:errorcluster)  [unwired: 15 in]
                n155 = for {
                  N: 15 -> [_]
                  tunnel: w220 -> [w231]
                  shift-right: [w235] -> w210
                  shift-left: w219 -> [w238]
                  tunnel: [w234] -> w212
                  i -> [w233]
                  n156 = Add(x=w233, y=2) -> (x+y=w229:i32)
                  n157 = case shown="2..12" w229 {
                    tunnel: [Pin_Mode."Output" ("Pin Mode (Input)") Pin_Mode."Output" ("Pin Mode (Input)") Pin_Mode."Output" ("Pin Mode (Input)") Pin_Mode."Input" ("Pin Mode (Input)") Pin_Mode."Output" ("Pin Mode (Input)")] -> w228
                    tunnel: [0 ("y") 1 ("y") 0 ("y") 0 ("y") 1 ("y")] -> w230
                    frame 0, Default {
                    }
                    frame 2..12 {
                    }
                    frame 13 {
                    }
                    frame 14 {
                    }
                    frame 15 {
                    }
                  }
                  n158 = call "Set Digital Pin Mode b.vi"("Arduino Resource in"=w231, "Digital I/O Pin"=w229, "Pin Mode (Input)"=w228, "error in"=w238) -> ("Arduino Resource out"=w237:T3, "error out"=w236:errorcluster)  [unwired: 10 in]
                  n159 = case shown="\"Output\"" w228 {
                    tunnel: w237 -> [w239 w246]
                    tunnel: w236 -> [w240 w245]
                    tunnel: [w240 w244] -> w235
                    tunnel: [w239 w243] -> w234
                    tunnel: w230 -> [_ w242]
                    tunnel: w229 -> [_ w241]
                    frame "Input", Default {
                    }
                    frame "Output" {
                      n160 = call "Digital Write Pin b.vi"("Arduino Resource in"=w246, "Digital I/O Pin (0)"=w241, "Value (0)"=w242, "error in"=w245) -> ("Arduino Resource out"=w243:T3, "error out"=w244:errorcluster)  [unwired: 10 in]
                    }
                  }
                }
                n161 = case shown="No Error" w210 {
                  tunnel: w212 -> [_ w226]
                  tunnel: ["Conexão estabelecida!" ("Mensagem") "Falha ao conectar!" ("Mensagem")] -> w211
                  frame No Error {
                    n162 = property on="Frames" class="TabCtl (strict)"("Value"=1 ("y")) -> ()  [unwired: 2 in, 2 out]
                  }
                  frame Error {
                    n163 = Unbundle By Name(w226) -> ("connection ID in"=w227:refnum<k31>)
                    n164 = TCP Close Connection(connection ID=w227) -> (error out=w225:errorcluster)  [unwired: 2 in, 1 out]
                    n165 = property on="Frames" class="TabCtl (strict)"("Value"=0 ("y")) -> ()  [unwired: 2 in, 2 out]
                    n166 = call <vilib>:"Clear Errors.vi"("error in (no error)"=w225) -> ()  [unwired: 5 in, 2 out]
                  }
                }
                n167 = local write "Arduino Resource out"(w212) -> ()
                n168 = property on="Mensagem" class="Str"("Value"=w211) -> ()  [unwired: 2 in, 2 out]
              }
              frame #3 {
                n169 = case shown="No Error" w257 {
                  frame No Error {
                    n170 = local read "Arduino Resource out"() -> (w259:T3)
                    n171 = stacked-sequence {
                      tunnel: w259 -> [w262 w266 w268 _ w271 w272 w276]
                      tunnel: 0.0 ("Capacitor:") -> [_ _ _ _ w270 _ _]
                      frame #0 {
                        # "DESLIGA BARRAMENTO"
                        n172 = call "Digital Write Pin b.vi"("Arduino Resource in"=w262, "Digital I/O Pin (0)"=u8 15, "Value (0)"=u8 1) -> ()  [unwired: 11 in, 2 out]
                      }
                      frame #1 {
                        # "LIGA RESITOR DE DESCARGA"
                        n173 = call "Digital Write Pin b.vi"("Arduino Resource in"=w266, "Digital I/O Pin (0)"=u8 11, "Value (0)"=u8 0) -> ()  [unwired: 11 in, 2 out]
                        n174 = property on="Mensagem" class="Str"("Value"="Descarregando Capacitores!" ("Mensagem")) -> ()  [unwired: 2 in, 2 out]
                      }
                      frame #2 {
                        n175 = call "SET_CAPACITOR.vi"("Arduino Resource in"=w268, "Capacitor"=408.8) -> ()  [unwired: 7 in, 2 out]
                      }
                      frame #3 {
                        # "AGUARDA DESCARGA"
                        n176 = Wait (ms)(milliseconds to wait=u32 3000) -> ()  [unwired: 1 out]
                      }
                      frame #4 {
                        # "AJUSTA VALOR DO CAPACITOR"
                        n177 = call "SET_CAPACITOR.vi"("Arduino Resource in"=w271, "Capacitor"=w270) -> ()  [unwired: 7 in, 2 out]
                      }
                      frame #5 {
                        # "DESLIGA RESISTOR DE DESCARGA"
                        n178 = call "Digital Write Pin b.vi"("Arduino Resource in"=w272, "Digital I/O Pin (0)"=u8 11, "Value (0)"=u8 1) -> ()  [unwired: 11 in, 2 out]
                      }
                      frame #6 {
                        # "LIGA BARRAMENTO DE MEDI敲O"
                        n179 = call "Digital Write Pin b.vi"("Arduino Resource in"=w276, "Digital I/O Pin (0)"=u8 15, "Value (0)"=u8 0) -> ()  [unwired: 11 in, 2 out]
                        n180 = property on="Mensagem" class="Str"("Value"="Conexão estabelecida!" ("Mensagem")) -> ()  [unwired: 2 in, 2 out]
                      }
                    }
                  }
                  frame Error {
                  }
                }
              }
            }
          }
          event "Capacitor:": Value Change {
            n181 = event-data() -> ()  [unwired: 1 in, 6 out]
            n182 = local write "ATUALIZAR CAP"(FALSE ("RESET TIMER")) -> ()
            n183 = local write "Mensagem"("Preparando para atualizar!" ("Mensagem")) -> ()
          }
          event "CALIBRA敲O": Value Change {
            n184 = event-data() -> ()  [unwired: 1 in, 6 out]
            n185 = local write "CAL"(TRUE) -> ()
            n186 = local write "Table"(string[][] [] ("Table")) -> ()
            n187 = local read "Arduino Resource out"() -> (w282:T3)
            n188 = stacked-sequence {
              tunnel: w282 -> [w287 w291 w293 _ w296 w297 w301]
              tunnel: 0.0 ("Capacitor:") -> [_ _ _ _ w295 _ _]
              frame #0 {
                # "DESLIGA BARRAMENTO"
                n189 = call "Digital Write Pin b.vi"("Arduino Resource in"=w287, "Digital I/O Pin (0)"=u8 15, "Value (0)"=u8 1) -> ()  [unwired: 11 in, 2 out]
              }
              frame #1 {
                # "LIGA RESITOR DE DESCARGA"
                n190 = call "Digital Write Pin b.vi"("Arduino Resource in"=w291, "Digital I/O Pin (0)"=u8 11, "Value (0)"=u8 0) -> ()  [unwired: 11 in, 2 out]
                n191 = property on="Mensagem" class="Str"("Value"="Descarregando Capacitores!" ("Mensagem")) -> ()  [unwired: 2 in, 2 out]
              }
              frame #2 {
                n192 = call "SET_CAPACITOR.vi"("Arduino Resource in"=w293, "Capacitor"=408.8) -> ()  [unwired: 7 in, 2 out]
              }
              frame #3 {
                # "AGUARDA DESCARGA"
                n193 = Wait (ms)(milliseconds to wait=u32 3000) -> ()  [unwired: 1 out]
              }
              frame #4 {
                # "AJUSTA VALOR DO CAPACITOR"
                n194 = call "SET_CAPACITOR.vi"("Arduino Resource in"=w296, "Capacitor"=w295) -> ()  [unwired: 7 in, 2 out]
              }
              frame #5 {
                # "DESLIGA RESISTOR DE DESCARGA"
                n195 = call "Digital Write Pin b.vi"("Arduino Resource in"=w297, "Digital I/O Pin (0)"=u8 11, "Value (0)"=u8 1) -> ()  [unwired: 11 in, 2 out]
              }
              frame #6 {
                # "LIGA BARRAMENTO DE MEDI敲O"
                n196 = call "Digital Write Pin b.vi"("Arduino Resource in"=w301, "Digital I/O Pin (0)"=u8 12, "Value (0)"=u8 0) -> ()  [unwired: 11 in, 2 out]
                n197 = property on="Mensagem" class="Str"("Value"="Calibrando!" ("Mensagem")) -> ()  [unwired: 2 in, 2 out]
              }
            }
          }
        }
        n198 = Or(x="SAIR", y="SAIR 2") -> (x .or. y?=w28:bool)
      }
    }
    frame #2 {
      n199 = local read "Arduino Resource out"() -> (w305:T3)
      n200 = Unbundle By Name(w305) -> ("connection ID in"=w304:refnum<k31>)
      n201 = TCP Close Connection(connection ID=w304) -> ()  [unwired: 2 in, 2 out]
    }
  }
